vi "start ROI set - CCD2.vi"(6 "Rectangle top CCD2":T1 {"Rotation" format="%.2f"; "Left" scale=0.0..1024.0; "Right" scale=0.0..1024.0}, 10 "Rectangle small CCD2":T1 {"Rotation" format="%.2f"; "Left" scale=0.0..1024.0; "Right" scale=0.0..1024.0}, 11 "Rectangle big CCD2":T1 {"Rotation" format="%.2f"; "Left" scale=0.0..1024.0; "Right" scale=0.0..1024.0}) -> (1 "ROI Descriptor top":T2={"Global Rectangle"=[1279, 916, 1775, 986], "Contours"=[{"ID"=enum."External", "Type"=12, "Coordinates"=[1280, 918, 1774, 984, 180289]}]} {"Contours"."Type" items=["No Selection", "Point", "Line", "Rectangle", "Oval", "Polygon", "Freehand Region", "Annulus", "Unused2", "Unused3", "Broken Line", "Freehand Line", "Rotated Rectangle"]}, 2 "ROI Descriptor (Small)":T2={"Global Rectangle"=[1279, 916, 1775, 986], "Contours"=[{"ID"=enum."External", "Type"=12, "Coordinates"=[1280, 918, 1774, 984, 180289]}]} {"Contours"."Type" items=["No Selection", "Point", "Line", "Rectangle", "Oval", "Polygon", "Freehand Region", "Annulus", "Unused2", "Unused3", "Broken Line", "Freehand Line", "Rotated Rectangle"]}, 3 "ROI Descriptor (big)":T2={"Global Rectangle"=[1279, 916, 1775, 986], "Contours"=[{"ID"=enum."External", "Type"=12, "Coordinates"=[1280, 918, 1774, 984, 180289]}]} {"Contours"."Type" items=["No Selection", "Point", "Line", "Rectangle", "Oval", "Polygon", "Freehand Region", "Annulus", "Unused2", "Unused3", "Broken Line", "Freehand Line", "Rotated Rectangle"]})   [LabVIEW 2017]
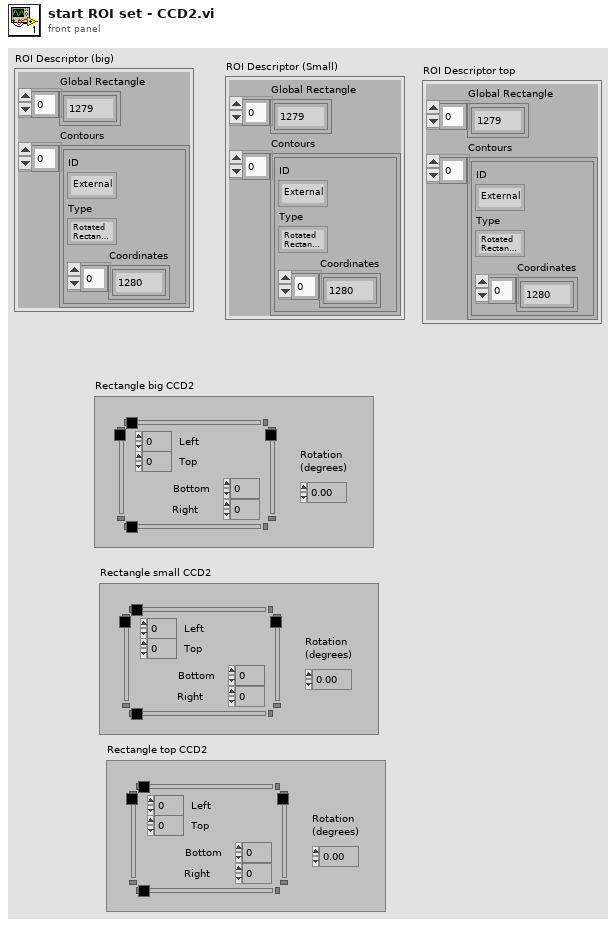
[diagram p1: front panel]
types:
  T1 = typedef "IMAQ Rectangle" = cluster{"Left":i32, "Top":i32, "Right":i32, "Bottom":i32, "Rotation":dbl}
  T2 = cluster{"Global Rectangle":i32[], "Contours":cluster{"ID":enum32{"External", "Internal"}, "Type":u32, "Coordinates":i32[]}[]}
  T3 = typedef "ROI Descriptor" = cluster{"Global Rectangle":i32[], "Contours":cluster{"ID":enum32{"External", "Internal"}, "Type":u32, "Coordinates":i32[]}[]}
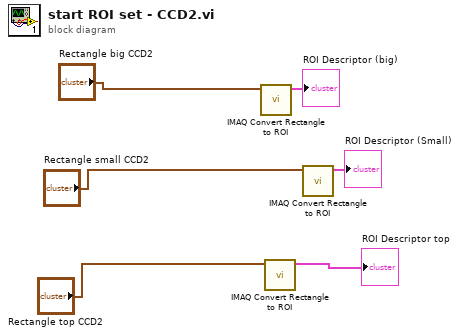
[diagram p0: block diagram]
diagram:
  n1 = call "IMAQ Convert Rectangle to ROI"("Rectangle"="Rectangle big CCD2") -> ("ROI Descriptor"=→"ROI Descriptor (big)":T3)  [unwired: 8 in, 1 out]
  n2 = call "IMAQ Convert Rectangle to ROI"("Rectangle"="Rectangle top CCD2") -> ("ROI Descriptor"=→"ROI Descriptor top":T3)  [unwired: 8 in, 1 out]
  n3 = call "IMAQ Convert Rectangle to ROI"("Rectangle"="Rectangle small CCD2") -> ("ROI Descriptor"=→"ROI Descriptor (Small)":T3)  [unwired: 8 in, 1 out]
